vi "z-transform.vi"(11 "input array":dbl[](array[numeric])) -> (3 "output array":dbl[](array[numeric]))   [LabVIEW 2013]
uses:
  <vilib>/Analysis/NI_AALBase.lvlib
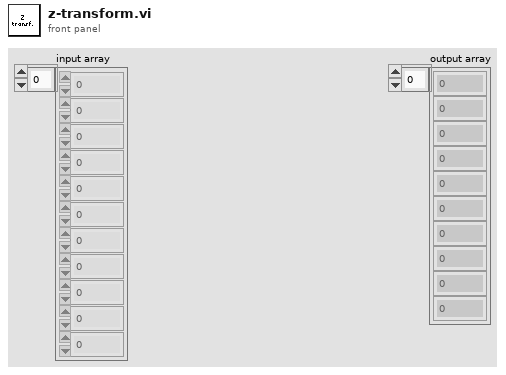
[diagram p1: front panel]
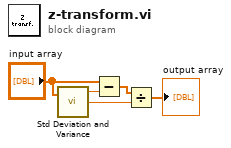
[diagram p0: block diagram]
diagram:
  n1 = call <vilib>:"Std Deviation and Variance.vi"("X"="input array") -> ("mean"=w4:dbl, "standard deviation"=w2:dbl)  [unwired: 1 in, 1 out]
  n2 = Subtract(x="input array", y=w4) -> (x-y=w3:dbl[])
  n3 = Divide(x=w3, y=w2) -> (x/y=→"output array":dbl[])
